vi "Main - Copy.vi"() -> ()   [LabVIEW 2018]
doc: "The myRIO Project template acquires acceleration data from the onboard accelerometer and displays the changes of acceleration values in a waveform chart."
uses:
  <vilib>/imath/engines/lvmath/Plug In/_Char/NIMS_CH_character datatype.ctl
  <vilib>/Analysis/coordinate.llb/2D Cartesian Coordinate Rotation (Scalar).vi
  <vilib>/myRIO/Common/Instrument Driver Framework/myRIO v1.0/UART/vis/myRIO v1.0 Close UART.vi
  <vilib>/robotics/Navigation/shared/WorldMap/OccupancyGridWorldMap/NI_Robotics_OccupancyGridWorldMap.lvclass
  C:/Program Files (x86)/National Instruments/LabVIEW 2018/vi.lib/robotics/Navigation/shared/WorldMap/AbstractWorldMap/NI_Robotics_AbstractWorldMap.lvclass
  <vilib>/robotics/Navigation/shared/MapNode/OccupancyGridNode/NI_Robotics_OccupancyGridMapNode.lvclass
  C:/Program Files (x86)/National Instruments/LabVIEW 2018/vi.lib/robotics/Navigation/shared/MapNode/AbstractAstarNode/NI_Robotics_AbstractAstarNode.lvclass
  <vilib>/imath/engines/lvmath2/RunTimeEngine/Managers/WorkSpace/UID Generator.vi
  <vilib>/imath/engines/lvmath/Plug In/_Char/NIMS_CH_String to Character Array.vi
  <vilib>/imath/engines/lvmath2/RunTimeEngine/IndexRead/NIMS V(S).vi
  <instcachedir>/0/NIMS V(S)_0488751826AF41519A22953C041130DC.lvgen/NIMS V(S)_0488751826AF41519A22953C041130DC_003.vi
  <vilib>/imath/engines/lvmath2/RunTimeEngine/RunTimeType/NIMS_RunTimeType_From StrictType (excl LVString).vi
  <instcachedir>/0/NIMS_RunTimeType_From StrictType (excl LVString)_E7E34A65C99947108168652BAD14964D.lvgen/NIMS_RunTimeType_From StrictType (excl LVString)_E7E34A65C99947108168652BAD14964D_000.vi
  <vilib>/imathl/engines/lvmath/Functions/Error Handling/Create Error.vi
  <vilib>/imath/engines/lvmath2/RunTimeEngine/LocalVariableDefStatement/MC_LocalVariableDefStatement_Display.vi
  <vilib>/imath/engines/lvmath2/RunTimeEngine/BuiltInFunctions/acos/NIMS_acos(C).vi
  <instcachedir>/0/NIMS_acos(C)_EB9F8BBCD4F84158BAE4AC9B979C42E8.lvgen/NIMS_acos(C)_EB9F8BBCD4F84158BAE4AC9B979C42E8_001.vi
  <vilib>/imath/engines/lvmath2/RunTimeEngine/Managers/SymbolTable/Clear UID.vi
  <vilib>/imath/engines/lvmath2/RunTimeEngine/NodeEndStatement/NIMS_NodeEndStatement_Output.vi
  <instcachedir>/0/NIMS_NodeEndStatement_Output_53EC0D466D134D7ABD903AC30B43404B.lvgen/NIMS_NodeEndStatement_Output_53EC0D466D134D7ABD903AC30B43404B_001.vi
  <instcachedir>/0/NIMS_NodeEndStatement_Output_53EC0D466D134D7ABD903AC30B43404B.lvgen/NIMS_NodeEndStatement_Output_53EC0D466D134D7ABD903AC30B43404B_011.vi
  <instcachedir>/0/NIMS_NodeEndStatement_Output_53EC0D466D134D7ABD903AC30B43404B.lvgen/NIMS_NodeEndStatement_Output_53EC0D466D134D7ABD903AC30B43404B_009.vi
  <vilib>/imath/engines/lvmath2/RunTimeEngine/ErrorHandling/NIMS_Finalize Error.vi
  <vilib>/imath/engines/lvmath2/RunTimeEngine/BuiltInFunctions/round/NIMS_round(DBL-S).vi
  <vilib>/imath/engines/lvmath2/RunTimeEngine/BuiltInFunctions/char/NIMS_char.vi
  <vilib>/imath/engines/lvmath/Plug In/_Char/NIMS_CH_String CV to Character 2D.vi
  <instcachedir>/0/NIMS_CH_String CV to Character 2D_831D8380D97041D793313BBAC4831DC8.lvgen/NIMS_CH_String CV to Character 2D_831D8380D97041D793313BBAC4831DC8_000.vi
  <instcachedir>/0/NIMS_RunTimeType_From StrictType (excl LVString)_E7E34A65C99947108168652BAD14964D.lvgen/NIMS_RunTimeType_From StrictType (excl LVString)_E7E34A65C99947108168652BAD14964D_001.vi
  <vilib>/imath/engines/lvmath2/RunTimeSupport/NIMS_Error if Not Equal.vi
  <instcachedir>/0/NIMS_Error if Not Equal_C77461FADD9B4AE6B0EA3ED6E3A6D94D.lvgen/NIMS_Error if Not Equal_C77461FADD9B4AE6B0EA3ED6E3A6D94D_000.vi
  <vilib>/imath/engines/lvmath2/RunTimeEngine/IndexReplace/NIMS M(S,S)=S.vi
  <instcachedir>/0/NIMS M(S,S)=S_5DAF17B45D8A4C8588C7CF468644990A.lvgen/NIMS M(S,S)=S_5DAF17B45D8A4C8588C7CF468644990A_002.vi
  <vilib>/imath/engines/lvmath2/RunTimeEngine/ErrorHandling/NIMS_Create Error From Enums.vi
  <vilib>/imath/engines/lvmath2/RunTimeEngine/RangeToken/NIMS_Range_R2 - Integer.vi
  <instcachedir>/0/NIMS_Range_R2 - Integer_E35B921DECF84AADB7325A02D418BFCC.lvgen/NIMS_Range_R2 - Integer_E35B921DECF84AADB7325A02D418BFCC_000.vi
  <vilib>/imath/engines/lvmath2/RunTimeEngine/CommandStatement/MC_CommandStatement_break.vi
  <vilib>/imath/engines/lvmath2/RunTimeEngine/BuiltInFunctions/min/2 inputs/NIMS_min(RG,RG)-no size check.vi
  <instcachedir>/0/NIMS_min(RG,RG)-no size check_7F67BAB91AFC452D9517D2EA1C8F5F88.lvgen/NIMS_min(RG,RG)-no size check_7F67BAB91AFC452D9517D2EA1C8F5F88_001.vi
  <vilib>/imath/engines/lvmath2/RunTimeEngine/BuiltInFunctions/max/2 inputs/NIMS_max(RG,RG)-no size check.vi
  <instcachedir>/0/NIMS_max(RG,RG)-no size check_F871939977644B7683C1350DCCAD7557.lvgen/NIMS_max(RG,RG)-no size check_F871939977644B7683C1350DCCAD7557_001.vi
  <vilib>/imath/engines/lvmath2/RunTimeEngine/IndexRead/NIMS M(S,S).vi
  <instcachedir>/0/NIMS M(S,S)_AC51E74150A542F7991B9634C66F3096.lvgen/NIMS M(S,S)_AC51E74150A542F7991B9634C66F3096_002.vi
  <instcachedir>/0/NIMS_min(RG,RG)-no size check_7F67BAB91AFC452D9517D2EA1C8F5F88.lvgen/NIMS_min(RG,RG)-no size check_7F67BAB91AFC452D9517D2EA1C8F5F88_002.vi
  <instcachedir>/0/NIMS_min(RG,RG)-no size check_7F67BAB91AFC452D9517D2EA1C8F5F88.lvgen/NIMS_min(RG,RG)-no size check_7F67BAB91AFC452D9517D2EA1C8F5F88_003.vi
  <vilib>/imath/engines/lvmath/Plug In/_Char/NIMS_CH_Character 2D to String 1D.vi
  <instcachedir>/0/NIMS_NodeEndStatement_Output_53EC0D466D134D7ABD903AC30B43404B.lvgen/NIMS_NodeEndStatement_Output_53EC0D466D134D7ABD903AC30B43404B_012.vi
  <instcachedir>/0/NIMS_NodeEndStatement_Output_53EC0D466D134D7ABD903AC30B43404B.lvgen/NIMS_NodeEndStatement_Output_53EC0D466D134D7ABD903AC30B43404B_013.vi
  <instcachedir>/0/NIMS_NodeEndStatement_Output_53EC0D466D134D7ABD903AC30B43404B.lvgen/NIMS_NodeEndStatement_Output_53EC0D466D134D7ABD903AC30B43404B_016.vi
  <vilib>/imath/engines/lvmath2/RunTimeEngine/VariableToken/NIMS_VariableToken_CondDefined.vi
  <instcachedir>/0/NIMS_VariableToken_CondDefined_BADDB804EBCA4B86883699DABD34B224.lvgen/NIMS_VariableToken_CondDefined_BADDB804EBCA4B86883699DABD34B224_004.vi
  <vilib>/imath/engines/lvmath/Functions/Error Handling/MergeErrorsWrapper.vi
  <vilib>/myRIO/Common/Instrument Driver Framework/Utilities/vis/FPGA Ref Manager.vi
  <vilib>/myRIO/Common/Instrument Driver Framework/myRIO v1.0/myRIO v1.0 Reset FPGA.vi
  <vilib>/myRIO/Common/Instrument Driver Framework/myRIO v1.0/IRQ/vis/myRIO v1.0 IRQ Info FGV.vi
  <vilib>/myRIO/Common/Instrument Driver Framework/myRIO v1.0/IRQ/vis/myRIO v1.0 Timer IRQ Info FGV.vi
  <vilib>/myRIO/Common/Instrument Driver Framework/myRIO v1.0/IRQ/vis/myRIO v1.0 ISR Agent.vi
  <vilib>/myRIO/Instrument Drivers/Utilities/Utilities.lvlib
  <vilib>/imath/engines/lvmath2/RunTimeEngine/Managers/SymbolTable/NIMS_WorkSpace.lvlib
  <vilib>/Analysis/NI_AALPro.lvlib
  <vilib>/robotics/Navigation/NI_Robotics_Navigation .lvlib
panel:
  out "field":i32[][](array[numeric])
  out "error out":errorcluster
  in  "stop":bool
  in  "Tab Control":enum32{"Main", "Settings"}(tab)
  out "Dist Finish":dbl
  out "Theta Finish":dbl
  out "Read Camera":bool
  out "Data":string
  out "Position":cluster{"X":dbl, "Y":dbl, "Theta":dbl}
  out "X Finish":string[](array[string])
  out "Y Finish":string[](array[string])
  out "y path":i32[](array[numeric])
  out "x path":i32[](array[numeric])
  out "G":i32[][](array[numeric])
  in  "Motor Controller ID#  (I2C Address)":u8=1 min=1 max=4
  in  "Motor Controller ID#  (I2C Address) 2":u8=2 min=1 max=4
  in  "Servo Controller ID#  (I2C Address) 3":u8=3 min=1 max=4
  in  "Controller myRIO MXP Port A/B":tag="A/I2C"
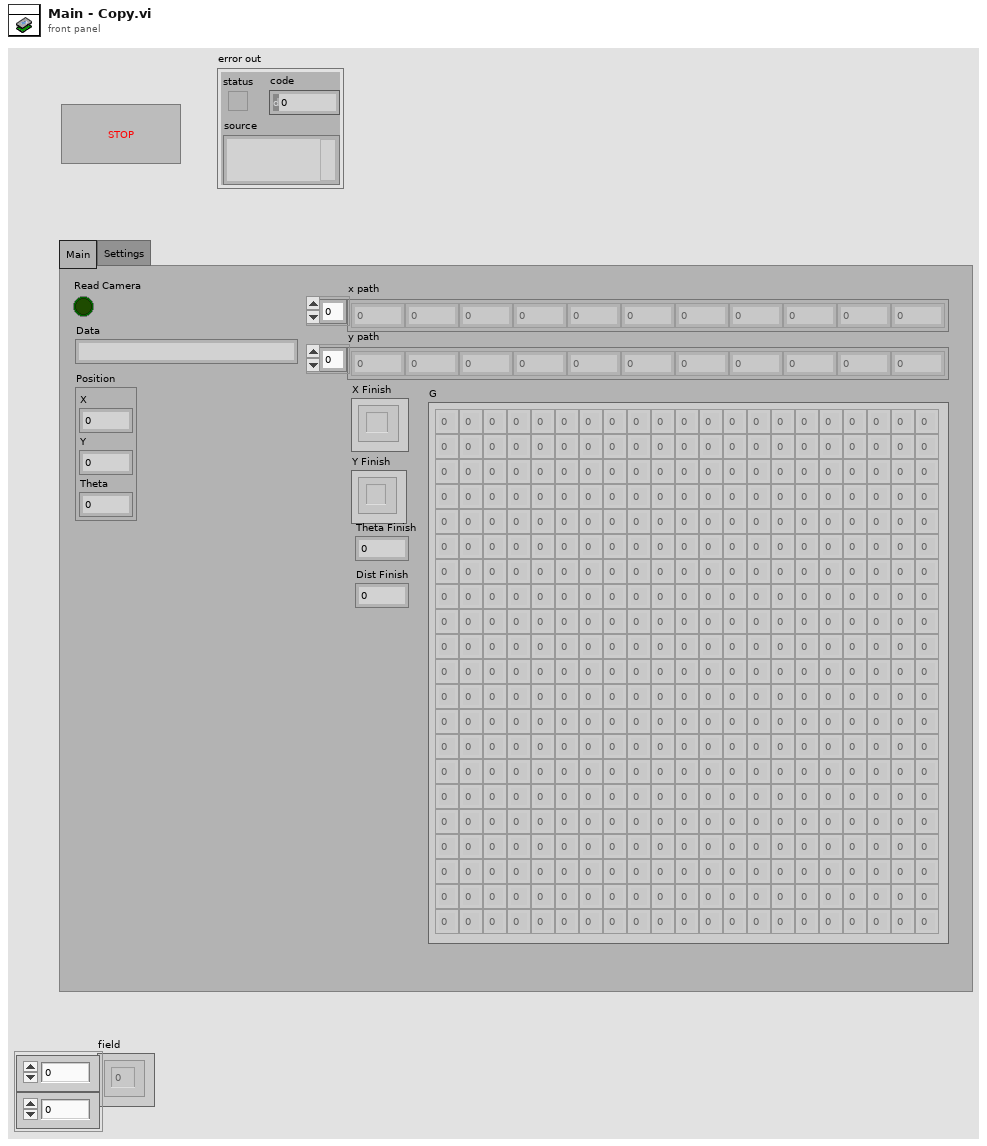
[diagram p1: front panel]
types:
  T1 = typedef "NIMS_CH_character datatype.ctl" = cluster{"Numeric":u8}
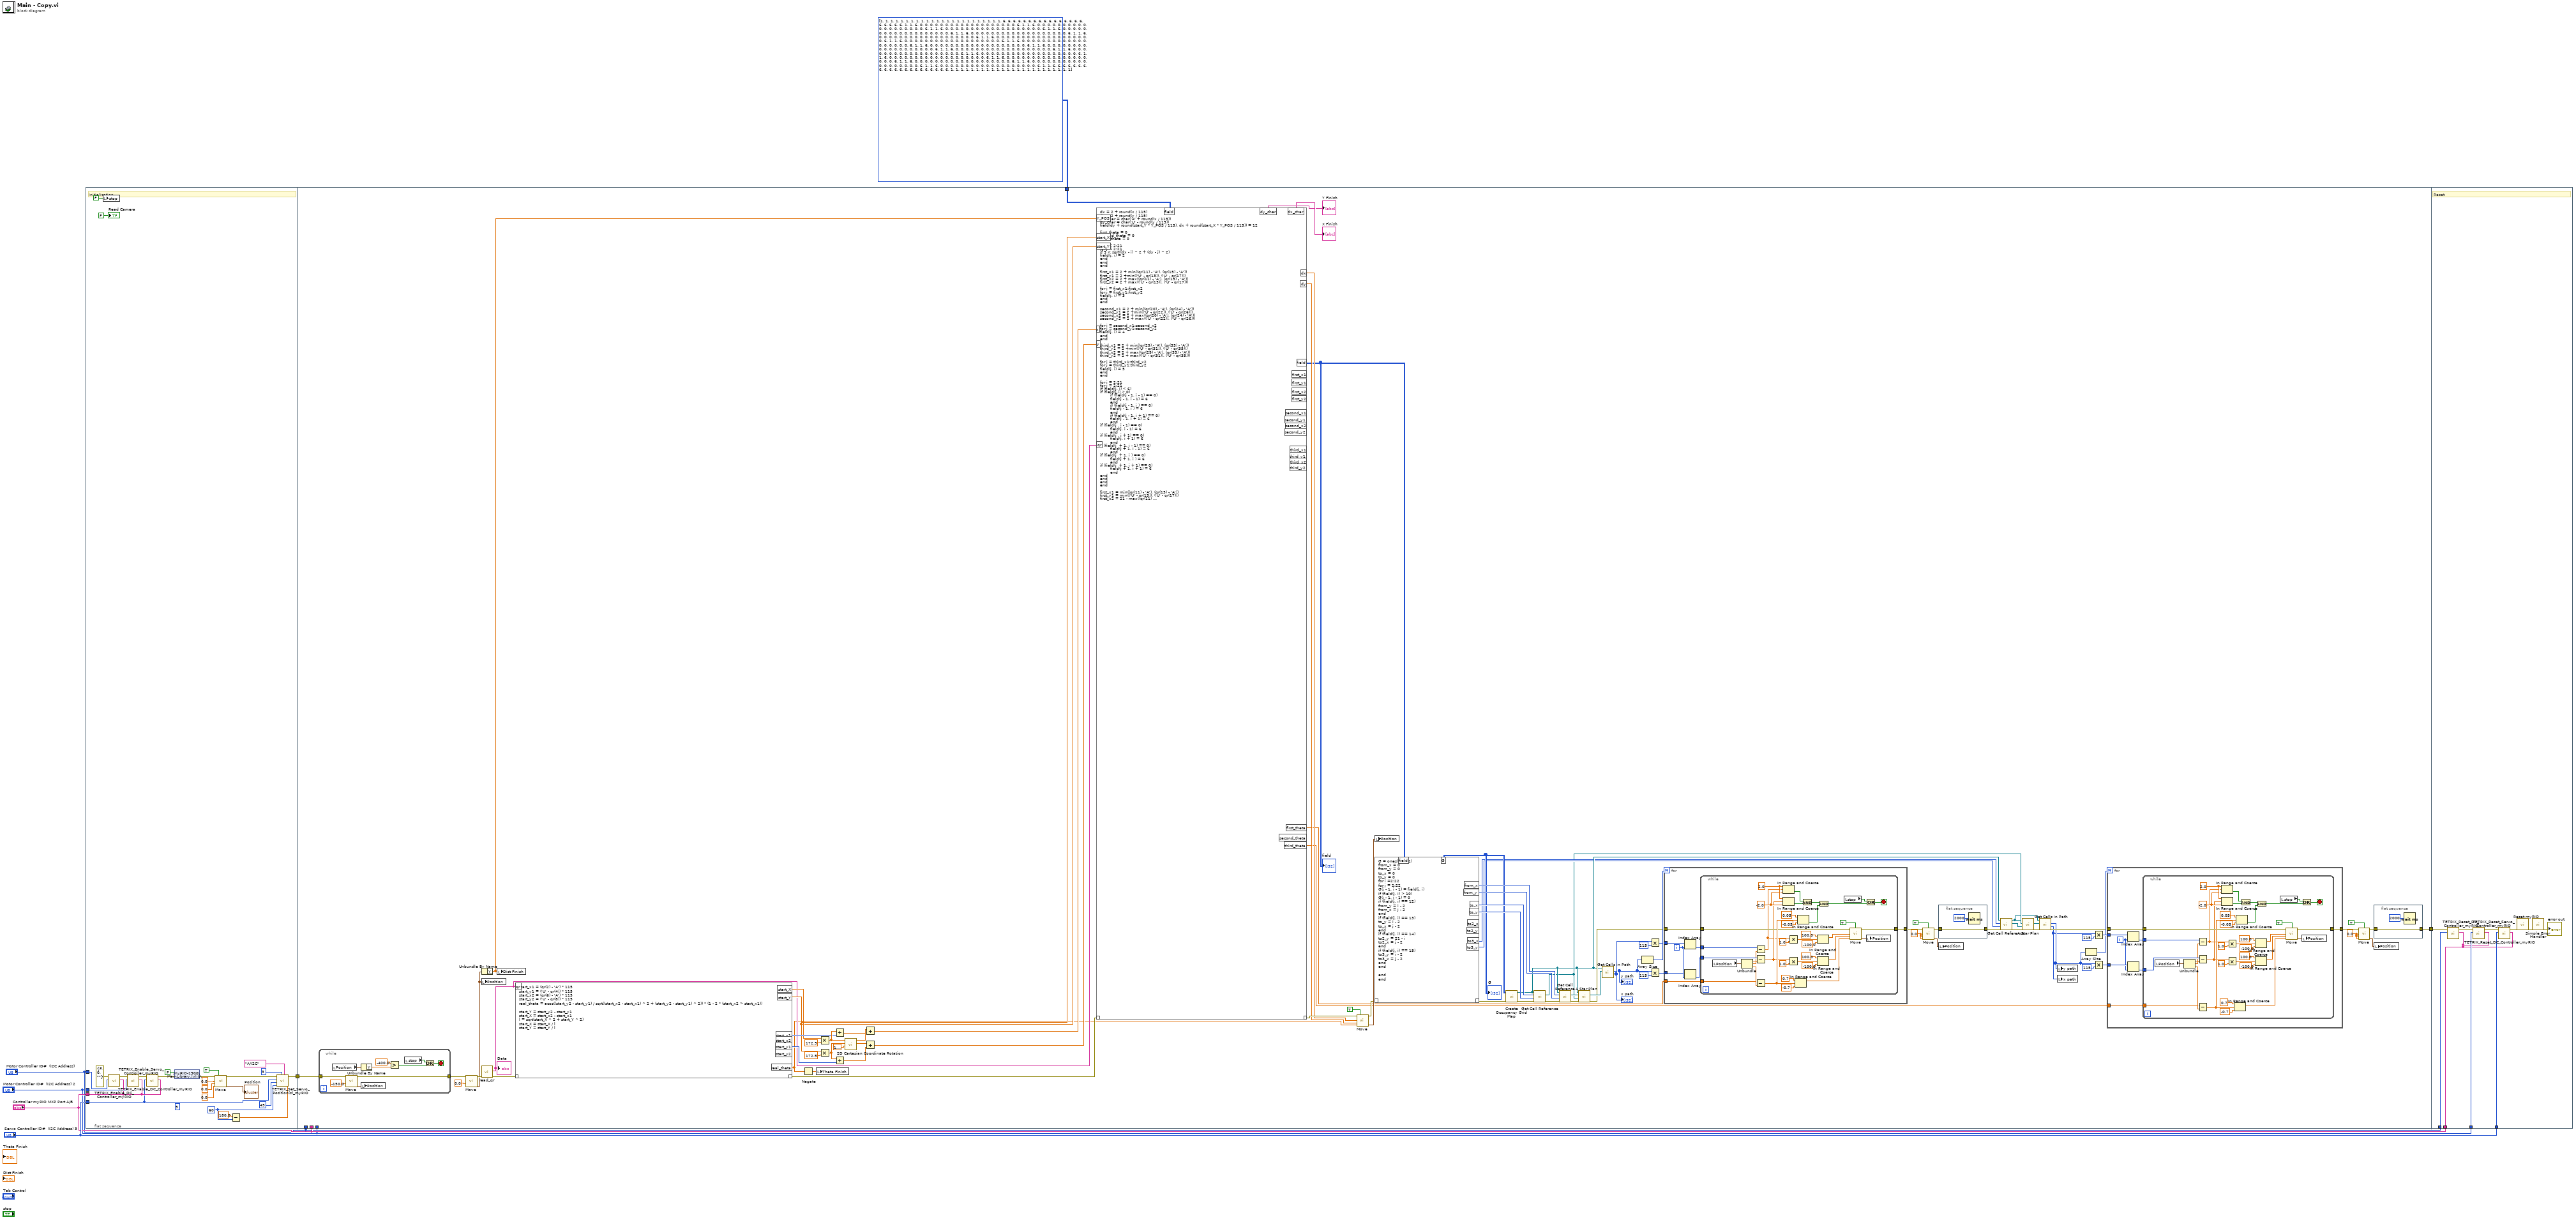
[diagram p0: block diagram]
diagram:
  n1 = flat-sequence {
    tunnel: "Motor Controller ID#  (I2C Address)" -> [w31]
    tunnel: "Motor Controller ID#  (I2C Address) 2" -> [w30]
    tunnel: "Controller myRIO MXP Port A/B" -> [w25]
    tunnel: "Servo Controller ID#  (I2C Address) 3" -> [w8]
    tunnel: [w9] -> w3
    tunnel: "Controller myRIO MXP Port A/B" -> [_]
    tunnel: "Motor Controller ID#  (I2C Address)" -> [_]
    tunnel: "Motor Controller ID#  (I2C Address) 2" -> [_]
    tunnel: w3 -> [w116]
    tunnel: u8[][] [[1, 1, 1, 1, 1, 1, 1, 1, 1, 1, 1, 1, 1, 1, 1, 1, 1, 1, 1, 1, 1, 1, 1], [1, 6, 6, 6, 6, 6, 6, 6, 6, 6, 6, 6, 6, 6, 6, 6, 6, 6, 6, 6, 6, 6, 1], [1, 6, 0, 0, 0, 0, 0, 0, 0, 0, 0, 0, 0, 0, 0, 0, 0, 0, 0, 0, 0, 6, 1], [1, 6, 0, 0, 0, 0, 0, 0, 0, 0, 0, 0, 0, 0, 0, 0, 0, 0, 0, 0, 0, 6, 1], [1, 6, 0, 0, 0, 0, 0, 0, 0, 0, 0, 0, 0, 0, 0, 0, 0, 0, 0, 0, 0, 6, 1], [1, 6, 0, 0, 0, 0, 0, 0, 0, 0, 0, 0, 0, 0, 0, 0, 0, 0, 0, 0, 0, 6, 1], [1, 6, 0, 0, 0, 0, 0, 0, 0, 0, 0, 0, 0, 0, 0, 0, 0, 0, 0, 0, 0, 6, 1], [1, 6, 0, 0, 0, 0, 0, 0, 0, 0, 0, 0, 0, 0, 0, 0, 0, 0, 0, 0, 0, 6, 1], [1, 6, 0, 0, 0, 0, 0, 0, 0, 0, 0, 0, 0, 0, 0, 0, 0, 0, 0, 0, 0, 6, 1], [1, 6, 0, 0, 0, 0, 0, 0, 0, 0, 0, 0, 0, 0, 0, 0, 0, 0, 0, 0, 0, 6, 1], [1, 6, 0, 0, 0, 0, 0, 0, 0, 0, 0, 0, 0, 0, 0, 0, 0, 0, 0, 0, 0, 6, 1], [1, 6, 0, 0, 0, 0, 0, 0, 0, 0, 0, 0, 0, 0, 0, 0, 0, 0, 0, 0, 0, 6, 1], [1, 6, 0, 0, 0, 0, 0, 0, 0, 0, 0, 0, 0, 0, 0, 0, 0, 0, 0, 0, 0, 6, 1], [1, 6, 0, 0, 0, 0, 0, 0, 0, 0, 0, 0, 0, 0, 0, 0, 0, 0, 0, 0, 0, 6, 1], [1, 6, 0, 0, 0, 0, 0, 0, 0, 0, 0, 0, 0, 0, 0, 0, 0, 0, 0, 0, 0, 6, 1], [1, 6, 0, 0, 0, 0, 0, 0, 0, 0, 0, 0, 0, 0, 0, 0, 0, 0, 0, 0, 0, 6, 1], [1, 6, 0, 0, 0, 0, 0, 0, 0, 0, 0, 0, 0, 0, 0, 0, 0, 0, 0, 0, 0, 6, 1], [1, 6, 0, 0, 0, 0, 0, 0, 0, 0, 0, 0, 0, 0, 0, 0, 0, 0, 0, 0, 0, 6, 1], [1, 6, 0, 0, 0, 0, 0, 0, 0, 0, 0, 0, 0, 0, 0, 0, 0, 0, 0, 0, 0, 6, 1], [1, 6, 0, 0, 0, 0, 0, 0, 0, 0, 0, 0, 0, 0, 0, 0, 0, 0, 0, 0, 0, 6, 1], [1, 6, 0, 0, 0, 0, 0, 0, 0, 0, 0, 0, 0, 0, 0, 0, 0, 0, 0, 0, 0, 6, 1], [1, 6, 6, 6, 6, 6, 6, 6, 6, 6, 6, 6, 6, 6, 6, 6, 6, 6, 6, 6, 6, 6, 1], [1, 1, 1, 1, 1, 1, 1, 1, 1, 1, 1, 1, 1, 1, 1, 1, 1, 1, 1, 1, 1, 1, 1]] ("Field") -> [w95]
    tunnel: [w40] -> w1
    tunnel: "Controller myRIO MXP Port A/B" -> [w4632]
    tunnel: "Motor Controller ID#  (I2C Address)" -> [w4636]
    tunnel: "Motor Controller ID#  (I2C Address) 2" -> [w4635]
    tunnel: "Servo Controller ID#  (I2C Address) 3" -> [w4633]
    tunnel: w1 -> [w4628]
    frame #0 {
      w15 = u8 60 ("Servo 4 Position (0 - 180 degrees)")
      (unwired) u8 5 ("Servo 1 Position (0 - 180 degrees)")
      # "Initialization"
      n2 = local write "stop"(FALSE ("Stop")) -> ()
      n3 = call <vilib>:"TETRIX_Enable_DC_Controller_myRIO.vi"("myRIO MXP Port A/B"=w25, "Controller ID#  (I2C Address)"=w31, "Error/Flow In"=errorcluster {"status"=FALSE, "code"=0, "source"=""}) -> ("Error/Flow Out"=w32:errorcluster)  [unwired: 4 in]
      n4 = call <vilib>:"TETRIX_Enable_DC_Controller_myRIO.vi"("myRIO MXP Port A/B"=w25, "Controller ID#  (I2C Address)"=w30, "Error/Flow In"=w32) -> ("Error/Flow Out"=w28:errorcluster)  [unwired: 4 in]
      n5 = call <vilib>:"TETRIX_Enable_Servo_Controller_myRIO.vi"("myRIO MXP Port A/B"=w25, "Controller ID#  (I2C Address)"=w8, "Error/Flow In"=w28) -> ("Error/Flow Out"=w27:errorcluster)  [unwired: 4 in]
      n6 = shared-variable "myRIO-1900\\MainLibrary.lvlib\\stop"(FALSE ("Stop"), error in=w27) -> (error out=w22:errorcluster)
      n7 = call "Move.vi"("Error/Flow In"=w22, "Reset"=TRUE, "x (mm/s)"=0.0, "y (mm/s)"=0.0, "theta (rad/s)"=0.0) -> ("Error/Flow Out"=w10:errorcluster, "Position"=→"Position":cluster{"X":dbl, "Y":dbl, "Theta":dbl})  [unwired: 9 in]
      n8 = Subtract(x=180.0, y=w15) -> (x-y=w14:dbl)
      n9 = call <vilib>:"TETRIX_Set_Servo_Position(s)_myRIO.vi"("Servo 4 Position (0 - 180 degrees)"=w14, "myRIO MXP Port A/B"=tag "A/I2C", "Controller ID#  (I2C Address)"=u8 3, "Servo 3 Position (0 - 180 degrees)"=w15, "Servo 2 Position (0 - 180 degrees)"=u8 45, "Servo 1 Position (0 - 180 degrees)"=w8, "Error/Flow In"=w10) -> ("Error/Flow Out"=w9:errorcluster)  [unwired: 2 in]
      "Read Camera" <- FALSE ("Read Camera")
    }
    frame #1 {
      w44 = 0.0 ("x (mm/s)")
      w79 = 0.0 ("x (mm/s)")
      n10 = while {
        tunnel: [w4623] -> w115
        tunnel: w116 -> [w4624]
        stop <- w4618 stop-if-true
        n11 = local read "Position"() -> (w4627:cluster{"X":dbl, "Y":dbl, "Theta":dbl})
        n12 = call "Move.vi"("Error/Flow In"=w4624, "y (mm/s)"=-150.0) -> ("Error/Flow Out"=w4623:errorcluster, "Position"=w4622:cluster{"X":dbl, "Y":dbl, "Theta":dbl})  [unwired: 12 in]
        n13 = Unbundle By Name(w4627) -> ("Y"=w4626:dbl)
        n14 = local write "Position"(w4622) -> ()
        n15 = Greater?(x=-400.0, y=w4626) -> (0:w4619:bool)
        n16 = local read "stop"() -> (w4620:bool)
        n17 = Or(x=w4620, y=w4619) -> (x .or. y?=w4618:bool)
      }
      n18 = call "Move.vi"("Error/Flow In"=w115, "y (mm/s)"=0.0) -> ("Error/Flow Out"=w117:errorcluster, "Position"=w96:cluster{"X":dbl, "Y":dbl, "Theta":dbl})  [unwired: 12 in]
      n19 = Unbundle By Name(w96) -> ("Y"=w37:dbl)
      n20 = local write "Position"(w96) -> ()
      n21 = call "read_qr.vi"("error in"=w117) -> ("error out"=w98:errorcluster, "Data"=w99:string)  [unwired: 8 in]
      "Data" <- w99
      n22 = local write "Dist Finish"(w37) -> ()
      n23 = mathscript code="start_x1 = (qr(2) - 'A') * 115\nstart_y1 = ('U' - qr(4)) * 115\nstart_x2 = (qr(6) - 'A') * 115\nstart_y2 = ('U' - qr(8)) * 115\nreal_theta = acos((start_y2 - start_y1) / sqrt((start_x2 - start_x1) ^ 2 + (start_y2 - start_y1) ^ 2)) * (1 - 2 * (start_x2 > start_x1))\n\nstart_Y = start_y2 - start_y1\nstart_X = start_x2 - start_x1\nl = sqrt(start_X ^ 2 + start_Y ^ 2)\nstart_X = start_X / l\nstart_Y = start_Y / l"("??"=w98, "qr"=w99) -> ("??"=w97:errorcluster, "real_theta"=w39:cdb, "start_x1"=w105:i32, "start_y1"=w104:i32, "start_X"=w103:dbl, "start_Y"=w102:dbl)  [unwired: 2 out]
      n24 = Negate(x=w39) -> (-x=w38:cdb)
      n25 = local write "Theta Finish"(w38) -> ()
      n26 = Multiply(x=w103, y=172.5) -> (x*y=w108:dbl)
      n27 = Multiply(x=w102, y=172.5) -> (x*y=w109:dbl)
      n28 = Add(x=w108, y=w105) -> (x+y=w110:dbl)
      n29 = Add(x=w109, y=w104) -> (x+y=w112:dbl)
      n30 = call-poly <vilib>:"2D Cartesian Coordinate Rotation.vi"("theta"=1.5707963267948966, "y"=w109, "x"=w108) -> ("y out"=w113:dbl, "x out"=w111:dbl)  [unwired: 6 in, 1 out]
      n31 = Add(x=w111, y=w110) -> (x+y=w101:dbl)
      n32 = Add(x=w113, y=w112) -> (x+y=w100:dbl)
      n33 = mathscript code="dx = 2 + round(x / 115)\ndy = 2 + round(y / 115)\ndx_char = char('A' + round(x / 115))\ndy_char = char('U' - round(y / 115))\nfield(dy + round(start_Y * Y_POS / 115), dx + round(start_X * Y_POS / 115)) = 12\n\nfirst_theta = 0\nsecond_theta = 0\nthird_theta = 0\n\nfor i = 2:21\nfor j = 2:21\nif 3 > sqrt((dx - i) ^ 2 + (dy - j) ^ 2)\nfield(j, i) = 2\nend\nend\nend\n\nfirst_x1 = 2 + min((qr(11) - 'A'), (qr(15) - 'A'))\nfirst_y1 = 2 +min(('U' - qr(13)), ('U' - qr(17)))\nfirst_x2 = 2 + max((qr(11) - 'A'), (qr(15) - 'A'))\nfirst_y2 = 2 + max(('U' - qr(13)), ('U' - qr(17)))\n\nfor i = first_x1:first_x2\nfor j = first_y1:first_y2\nfield(j, i) = 3\nend\nend\n\nsecond_x1 = 2 + min((qr(20) - 'A'), (qr(24) - 'A'))\nsecond_y1 = 2 +min(('U' - qr(22)), ('U' - qr(26)))\nsecond_x2 = 2 + max((qr(20) - 'A'), (qr(24) - 'A'))\nsecond_y2 = 2 + max(('U' - qr(22)), ('U' - qr(26)))\n\nfor i = second_x1:second_x2\nfor j = second_y1:second_y2\nfield(j, i) = 4\nend\nend\n\nthird_x1 = 2 + min((qr(29) - 'A'), (qr(33) - 'A'))\nthird_y1 = 2 +min(('U' - qr(31)), ('U' - qr(35)))\nthird_x2 = 2 + max((qr(29) - 'A'), (qr(33) - 'A'))\nthird_y2 = 2 + max(('U' - qr(31)), ('U' - qr(35)))\n\nfor i = third_x1:third_x2\nfor j = third_y1:third_y2\nfield(j, i) = 5\nend\nend\n\nfor i = 2:21\nfor j = 2:21\nif (field(j, i) < 6)\nif (field(j,i) > 0)\n        if (field(j - 1, i - 1) == 0)\n        field(j - 1, i - 1) = 6\n        end\n        if (field(j - 1, i ) == 0)\n        field(j - 1, i ) = 6\n        end\n        if (field(j - 1, i + 1) == 0)\n        field(j - 1, i + 1) = 6\n        end\nif (field(j , i - 1) == 0)\n        field(j, i - 1) = 6\n        end\nif (field(j , i + 1) == 0)\n        field(j, i + 1) = 6\n        end\nif (field(j  + 1, i - 1) == 0)\n        field(j + 1, i - 1) = 6\n        end\nif (field(j  + 1, i ) == 0)\n        field(j + 1, i ) = 6\n        end\nif (field(j  + 1, i + 1) == 0)\n        field(j + 1, i + 1) = 6\n        end\nend\nend\nend\nend\n\nfirst_x1 = min((qr(11) - 'A'), (qr(15) - 'A'))\nfirst_y1 = min(('U' - qr(13)), ('U' - qr(17)))\nfirst_x2 = 21 - max((qr(11) - 'A'), (qr(15) - 'A'))\nfirst_y2 = 21 - max(('U' - qr(13)), ('U' - qr(17)))\n\nmin_dist = min(first_x1, min(first_x2, min(first_y1, first_y2)))\nif min_dist == first_x1\n    field(2 + first_y1 + 1, 2 + 21 -first_x2 + 2) = 13\n    first_theta = pi / 2\nend\nif min_dist == first_x2\n    field(2 + first_y1 + 1, 2 + first_x1 - 2) = 13\n    first_theta = -pi / 2\nend\nif min_dist == first_y1\n    field(2 + 21 - first_y2 + 2, 2 + first_x1 + 1) = 13\n    first_theta = 0\nend\nif min_dist == first_y2\n    field(2 + first_y1 - 2, 2 + first_x1 + 1) = 13\n    first_theta = pi\nend\n\nfirst_x1 = min((qr(20) - 'A'), (qr(24) - 'A'))\nfirst_y1 = min(('U' - qr(22)), ('U' - qr(26)))\nfirst_x2 = 21 - max((qr(20) - 'A'), (qr(24) - 'A'))\nfirst_y2 = 21 - max(('U' - qr(22)), ('U' - qr(26)))\n\nmin_dist = min(first_x1, min(first_x2, min(first_y1, first_y2)))\nif min_dist == first_x1\n    field(2 + first_y1 + 1, 2 + 21 -first_x2 + 2) = 14\n    second_theta = pi / 2\nend\nif min_dist == first_x2\n    field(2 + first_y1 + 1, 2 + first_x1 - 2) = 14\n    second_theta = -pi / 2\nend\nif min_dist == first_y1\n    field(2 + 21 - first_y2 + 2, 2 + first_x1 + 1) = 14\n    second_theta = 0\nend\nif min_dist == first_y2\n    field(2 + first_y1 - 2, 2 + first_x1 + 1) = 14\n    second_theta = pi\nend\n\nfirst_x1 = min((qr(29) - 'A'), (qr(33) - 'A'))\nfirst_y1 = min(('U' - qr(31)), ('U' - qr(35)))\nfirst_x2 = 21 - max((qr(29) - 'A'), (qr(33) - 'A'))\nfirst_y2 = 21 - max(('U' - qr(31)), ('U' - qr(35)))\n\nmin_dist = min(first_x1, min(first_x2, min(first_y1, first_y2)))\nif min_dist == first_x1\n    field(2 + first_y1 + 1, 2 + 21 -first_x2 + 2) = 15\n    third_theta = pi / 2\nend\nif min_dist == first_x2\n    field(2 + first_y1 + 1, 2 + first_x1 - 2) = 15\n    third_theta = -pi / 2\nend\nif min_dist == first_y1\n    field(2 + 21 - first_y2 + 2, 2 + first_x1 + 1) = 15\n    third_theta = 0\nend\nif min_dist == first_y2\n    field(2 + first_y1 - 2, 2 + first_x1 + 1) = 15\n    third_theta = pi\nend\n\ndx = dx - 2\ndy = dy - 2\ndx = (x + start_X * Y_POS)\ndy = (y + start_Y * Y_POS)\ndx_char = char('A' + round(dx / 115))\ndy_char = char('U' - round(dy / 115))"("??"=w97, "x"=w101, "y"=w100, "field"=w95, "qr"=w99, "start_X"=w103, "start_Y"=w102, "Y_POS"=w37) -> ("??"=w92:errorcluster, "dx"=w90:dbl, "dy"=w89:dbl, "field"=w63:i32[][], "dx_char"=→"X Finish":string[], "dy_char"=→"Y Finish":string[], "first_theta"=w34:dbl, "third_theta"=w33:dbl)  [unwired: 13 out]
      "field" <- w63
      n34 = call "Move.vi"("Error/Flow In"=w92, "Reset"=TRUE, "x (mm/s)"=w90, "y (mm/s)"=w89, "theta (rad/s)"=w39) -> ("Error/Flow Out"=w82:errorcluster, "Position"=w88:cluster{"X":dbl, "Y":dbl, "Theta":dbl})  [unwired: 9 in]
      n35 = local write "Position"(w88) -> ()
      n36 = mathscript code="G = ones(21, 21)\nfrom_x = 0\nfrom_y = 0\nto_x = 0\nto_y = 0\nfor i =2:22\nfor j = 2:22\nG(j - 1, i - 1) = field(j, i)\nif (field(j, i) > 10)\nG(j - 1, i - 1) = 0\nif (field(j, i) == 12)\nfrom_y = i - 2\nfrom_x = j - 2\nend\nif (field(j, i) == 13)\nto_y = i - 2\nto_x = j - 2\nend\nif (field(j, i) == 14)\nto2_y = 21 - i\nto2_x = j - 2\nend\nif (field(j, i) == 15)\nto3_y = i - 2\nto3_x = j - 2\nend\nend\n\nend\nend"("??"=w82, "field"=w63) -> ("??"=w85:errorcluster, "from_x"=w84:i32, "from_y"=w83:i32, "to_x"=w65:i32, "to_y"=w64:i32, "to3_x"=w59:i32, "to3_y"=w58:i32, "G"=w62:i32[][])  [unwired: 2 out]
      "G" <- w62
      n37 = call <vilib>:"Create Occupancy Grid Map.vi"("error in (no error)"=w85, "occupancy grid"=w62) -> ("error out"=w68:errorcluster, "map reference out"=w60:refnum<data-value>)  [unwired: 8 in]
      n38 = call <vilib>:"Get Cell Reference.vi"("error in (no error)"=w68, "y"=w64, "x"=w65, "map reference in"=w60) -> ("error out"=w67:errorcluster, "cell reference"=w56:refnum<data-value>)  [unwired: 4 in, 2 out]
      n39 = call <vilib>:"Get Cell Reference.vi"("error in (no error)"=w67, "y"=w83, "x"=w84, "map reference in"=w60) -> ("error out"=w66:errorcluster, "cell reference"=w87:refnum<data-value>)  [unwired: 4 in, 2 out]
      n40 = call <vilib>:"A Star Plan.vi"("error in (no error)"=w66, "goal reference"=w56, "start reference"=w87, "map reference in"=w60) -> ("error out"=w71:errorcluster, "path references"=w86:refnum<data-value>[])  [unwired: 4 in, 2 out]
      n41 = call <vilib>:"Get Cells in Path.vi"("path references"=w86, "map reference in"=w60) -> ("y coordinates"=w76:i32[], "x coordinates"=w75:i32[])  [unwired: 6 in, 2 out]
      "y path" <- w75
      "x path" <- w76
      n42 = Array Size(array=w75) -> (size(s)=w74:i32)
      n43 = Multiply(x=w76, y=115) -> (x*y=w72:i32[])
      n44 = Multiply(x=w75, y=115) -> (x*y=w73:i32[])
      n45 = for {
        N: w74 -> [_]
        tunnel: w73 -> [w176]
        tunnel: w72 -> [w175]
        tunnel: w71 -> [w171]
        tunnel: [w170] -> w70
        tunnel: w34 -> [w169]
        i -> [w174]
        n46 = Index Array(array=w175, index=w174) -> (element=w172:i32)
        n47 = Index Array(array=w176, index=w174) -> (element=w173:i32)
        n48 = while {
          tunnel: w173 -> [w211]
          tunnel: w172 -> [w210]
          tunnel: w171 -> [w191]
          tunnel: [w190] -> w170
          tunnel: w169 -> [w177]
          stop <- w179 stop-if-true
          w207 = -2.0 ("lower limit")
          w208 = 2.0 ("upper limit")
          n49 = local read "Position"() -> (w214:cluster{"X":dbl, "Y":dbl, "Theta":dbl})
          n50 = Unbundle(w214) -> ("X"=w209:dbl, "Y"=w212:dbl, "Theta"=w213:dbl)
          n51 = Subtract(x=w210, y=w209) -> (x-y=w182:dbl)
          n52 = Subtract(x=w211, y=w212) -> (x-y=w186:dbl)
          n53 = Subtract(x=w177, y=w213) -> (x-y=w194:dbl)
          n54 = In Range and Coerce(upper limit=w208, x=w182, lower limit=w207) -> (In Range?=w206:bool)  [unwired: 1 out]
          n55 = In Range and Coerce(upper limit=w208, x=w186, lower limit=w207) -> (In Range?=w205:bool)  [unwired: 1 out]
          n56 = Multiply(x=w182, y=1.0) -> (x*y=w181:dbl)
          n57 = Multiply(x=w186, y=1.0) -> (x*y=w184:dbl)
          n58 = In Range and Coerce(upper limit=0.7, x=w194, lower limit=-0.7 ("upper limit")) -> (coerced(x)=w192:dbl)  [unwired: 1 out]
          n59 = In Range and Coerce(upper limit=0.05, x=w194, lower limit=-0.05) -> (In Range?=w202:bool)  [unwired: 1 out]
          n60 = And(x=w206, y=w205) -> (x .and. y?=w201:bool)
          n61 = In Range and Coerce(upper limit=100.0, x=w181, lower limit=-100.0 ("upper limit")) -> (coerced(x)=w188:dbl)  [unwired: 1 out]
          n62 = In Range and Coerce(upper limit=100.0, x=w184, lower limit=-100.0 ("upper limit")) -> (coerced(x)=w187:dbl)  [unwired: 1 out]
          n63 = And(x=w201, y=w202) -> (x .and. y?=w180:bool)
          n64 = local read "stop"() -> (w178:bool)
          n65 = call "Move.vi"("Error/Flow In"=w191, "Relative to Global Frame"=TRUE, "x (mm/s)"=w188, "y (mm/s)"=w187, "theta (rad/s)"=w192) -> ("Error/Flow Out"=w190:errorcluster, "Position"=w189:cluster{"X":dbl, "Y":dbl, "Theta":dbl})  [unwired: 9 in]
          n66 = Or(x=w178, y=w180) -> (x .or. y?=w179:bool)
          n67 = local write "Position"(w189) -> ()
        }
      }
      n68 = call "Move.vi"("Error/Flow In"=w70, "Relative to Global Frame"=TRUE, "x (mm/s)"=w79, "y (mm/s)"=w79, "theta (rad/s)"=w79) -> ("Error/Flow Out"=w69:errorcluster, "Position"=w80:cluster{"X":dbl, "Y":dbl, "Theta":dbl})  [unwired: 9 in]
      n69 = flat-sequence {
        tunnel: w69 -> [w167]
        tunnel: [w167] -> w61
        frame #0 {
          n70 = Wait (ms)(milliseconds to wait=u32 2000) -> ()  [unwired: 1 out]
        }
      }
      n71 = local write "Position"(w80) -> ()
      n72 = call <vilib>:"Get Cell Reference.vi"("error in (no error)"=w61, "y"=w58, "x"=w59, "map reference in"=w60) -> ("error out"=w57:errorcluster, "cell reference"=w55:refnum<data-value>, "map reference out"=w53:refnum<data-value>)  [unwired: 4 in, 1 out]
      n73 = call <vilib>:"A Star Plan.vi"("error in (no error)"=w57, "goal reference"=w55, "start reference"=w56, "map reference in"=w53) -> ("error out"=w54:errorcluster, "path references"=w52:refnum<data-value>[])  [unwired: 4 in, 2 out]
      n74 = call <vilib>:"Get Cells in Path.vi"("error in (no error)"=w54, "path references"=w52, "map reference in"=w53) -> ("error out"=w41:errorcluster, "y coordinates"=w35:i32[], "x coordinates"=w36:i32[])  [unwired: 5 in, 1 out]
      n75 = local write "y path"(w36) -> ()
      n76 = local write "x path"(w35) -> ()
      n77 = Array Size(array=w36) -> (size(s)=w47:i32)
      n78 = Multiply(x=w35, y=115) -> (x*y=w49:i32[])
      n79 = Multiply(x=w36, y=115) -> (x*y=w48:i32[])
      n80 = for {
        N: w47 -> [_]
        tunnel: w48 -> [w128]
        tunnel: w49 -> [w127]
        tunnel: w41 -> [w123]
        tunnel: [w122] -> w50
        tunnel: w33 -> [w121]
        i -> [w126]
        n81 = Index Array(array=w127, index=w126) -> (element=w124:i32)
        n82 = Index Array(array=w128, index=w126) -> (element=w125:i32)
        n83 = while {
          tunnel: w125 -> [w163]
          tunnel: w124 -> [w162]
          tunnel: w123 -> [w143]
          tunnel: [w142] -> w122
          tunnel: w121 -> [w129]
          stop <- w130 stop-if-true
          w159 = -2.0 ("lower limit")
          w160 = 2.0 ("upper limit")
          n84 = local read "Position"() -> (w166:cluster{"X":dbl, "Y":dbl, "Theta":dbl})
          n85 = Unbundle(w166) -> ("X"=w161:dbl, "Y"=w164:dbl, "Theta"=w165:dbl)
          n86 = Subtract(x=w162, y=w161) -> (x-y=w134:dbl)
          n87 = Subtract(x=w163, y=w164) -> (x-y=w138:dbl)
          n88 = Subtract(x=w129, y=w165) -> (x-y=w146:dbl)
          n89 = In Range and Coerce(upper limit=w160, x=w134, lower limit=w159) -> (In Range?=w158:bool)  [unwired: 1 out]
          n90 = In Range and Coerce(upper limit=w160, x=w138, lower limit=w159) -> (In Range?=w157:bool)  [unwired: 1 out]
          n91 = Multiply(x=w134, y=1.0) -> (x*y=w133:dbl)
          n92 = Multiply(x=w138, y=1.0) -> (x*y=w136:dbl)
          n93 = In Range and Coerce(upper limit=0.7, x=w146, lower limit=-0.7 ("upper limit")) -> (coerced(x)=w144:dbl)  [unwired: 1 out]
          n94 = In Range and Coerce(upper limit=0.05, x=w146, lower limit=-0.05) -> (In Range?=w154:bool)  [unwired: 1 out]
          n95 = And(x=w158, y=w157) -> (x .and. y?=w153:bool)
          n96 = In Range and Coerce(upper limit=100.0, x=w133, lower limit=-100.0 ("upper limit")) -> (coerced(x)=w140:dbl)  [unwired: 1 out]
          n97 = In Range and Coerce(upper limit=100.0, x=w136, lower limit=-100.0 ("upper limit")) -> (coerced(x)=w139:dbl)  [unwired: 1 out]
          n98 = And(x=w153, y=w154) -> (x .and. y?=w131:bool)
          n99 = local read "stop"() -> (w132:bool)
          n100 = call "Move.vi"("Error/Flow In"=w143, "Relative to Global Frame"=TRUE, "x (mm/s)"=w140, "y (mm/s)"=w139, "theta (rad/s)"=w144) -> ("Error/Flow Out"=w142:errorcluster, "Position"=w141:cluster{"X":dbl, "Y":dbl, "Theta":dbl})  [unwired: 9 in]
          n101 = Or(x=w132, y=w131) -> (x .or. y?=w130:bool)
          n102 = local write "Position"(w141) -> ()
        }
      }
      n103 = call "Move.vi"("Error/Flow In"=w50, "Relative to Global Frame"=TRUE, "x (mm/s)"=w44, "y (mm/s)"=w44, "theta (rad/s)"=w44) -> ("Error/Flow Out"=w51:errorcluster, "Position"=w43:cluster{"X":dbl, "Y":dbl, "Theta":dbl})  [unwired: 9 in]
      n104 = flat-sequence {
        tunnel: w51 -> [w119]
        tunnel: [w119] -> w40
        frame #0 {
          n105 = Wait (ms)(milliseconds to wait=u32 2000) -> ()  [unwired: 1 out]
        }
      }
      n106 = local write "Position"(w43) -> ()
    }
    frame #2 {
      # "Reset"
      n107 = call <vilib>:"TETRIX_Reset_DC_Controller_myRIO.vi"("myRIO MXP Port A/B"=w4632, "Controller ID#  (I2C Address)"=w4636, "Error/Flow In"=w4628) -> ("Error/Flow Out"=w4637:errorcluster)  [unwired: 4 in]
      n108 = call <vilib>:"TETRIX_Reset_DC_Controller_myRIO.vi"("myRIO MXP Port A/B"=w4632, "Controller ID#  (I2C Address)"=w4635, "Error/Flow In"=w4637) -> ("Error/Flow Out"=w4634:errorcluster)  [unwired: 4 in]
      n109 = call <vilib>:"TETRIX_Reset_Servo_Controller_myRIO.vi"("myRIO MXP Port A/B"=w4632, "Controller ID#  (I2C Address)"=w4633, "Error/Flow In"=w4634) -> ("Error/Flow Out"=w4631:errorcluster)  [unwired: 4 in]
      n110 = call <vilib>:"Reset myRIO.vi"("error in (no error)"=w4631) -> ("error out"=w4630:errorcluster)  [unwired: 10 in]
      n111 = call <vilib>:"Simple Error Handler.vi"("error in (no error)"=w4630) -> ("error out"=→"error out":errorcluster)  [unwired: 4 in, 4 out]
    }
  }
